vi "Check Descriptor.vi"(11 "Descriptor":string) -> (0 "error out":errorcluster, 1 "Reason":string, 2 "Ok":bool, 3 "Descriptor out":string)   [LabVIEW 2015]
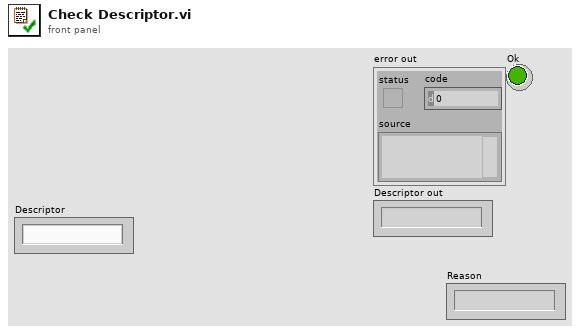
[diagram p1: front panel]
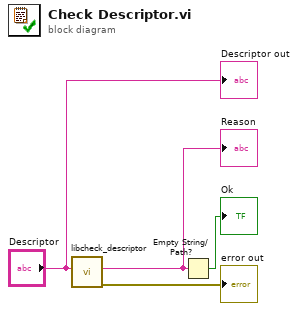
[diagram p0: block diagram]
diagram:
  n1 = call "libcheck_descriptor.vi"("Descriptor"="Descriptor") -> ("error out"=→"error out":errorcluster, "result"=w2:string)  [unwired: 9 in]
  "Reason" <- w2
  n2 = Empty String/Path?(string/path=w2) -> (empty?=→"Ok":bool)
  "Descriptor out" <- "Descriptor"
